vi "SampleSubVI.vi"(0 "task out":refnum<k21> caption="任务输出", 1 "Courter 1":refnum<k21> caption="任务/通道输入1", 3 "Courter 4":refnum<k21> caption="任务/通道输入4", 4 "Courter 2":refnum<k21> caption="任务/通道输入2", 6 "数组":sgl[](array[numeric]), 10 "Courter 3":refnum<k21> caption="任务/通道输入3", 11 "Courter 7":refnum<k21> caption="任务/通道输入7", 15 "Courter 5":refnum<k21> caption="任务/通道输入5", 19 "Courter 8":refnum<k21> caption="任务/通道输入8", 23 "Courter 6":refnum<k21> caption="任务/通道输入6") -> (5 "加速度信号2":dbl[](array[numeric]), 7 "压力信号":dbl[](array[numeric]), 8 "轴向位移":dbl[](array[numeric]), 9 "轴向力":dbl[](array[numeric]), 12 "vmic反馈数据":sgl[](array[numeric]), 13 "力臂":dbl[](array[numeric]), 14 "AngleSample":dbl[](array[numeric]), 16 "加速度信号":dbl[](array[numeric]), 17 "同步信号":dbl[](array[numeric]), 18 "AngleSample 2":dbl[](array[numeric]), 20 "ForceSampledata":dbl[](array[numeric]), 21 "F_outrange":bool[](array[boolean]), 24 "error out":errorcluster, 25 "PositionSampleData":dbl[](array[numeric]), 27 "TorqueSample":dbl[](array[numeric]))   [LabVIEW 2014]
uses:
  <vilib>/DAQmx/read.llb/DAQmx Read (Analog 1D DBL NChan 1Samp).vi
  <vilib>/DAQmx/read.llb/DAQmx Read (Counter DBL 1Chan 1Samp).vi
panel:
  out "ACC1 4":dbl
  out "ACC1 3":dbl
  out "ACC1 2":dbl
  out "ACC1":dbl
  out "data":dbl[](array[numeric]) caption="数据" format="%0.2f"
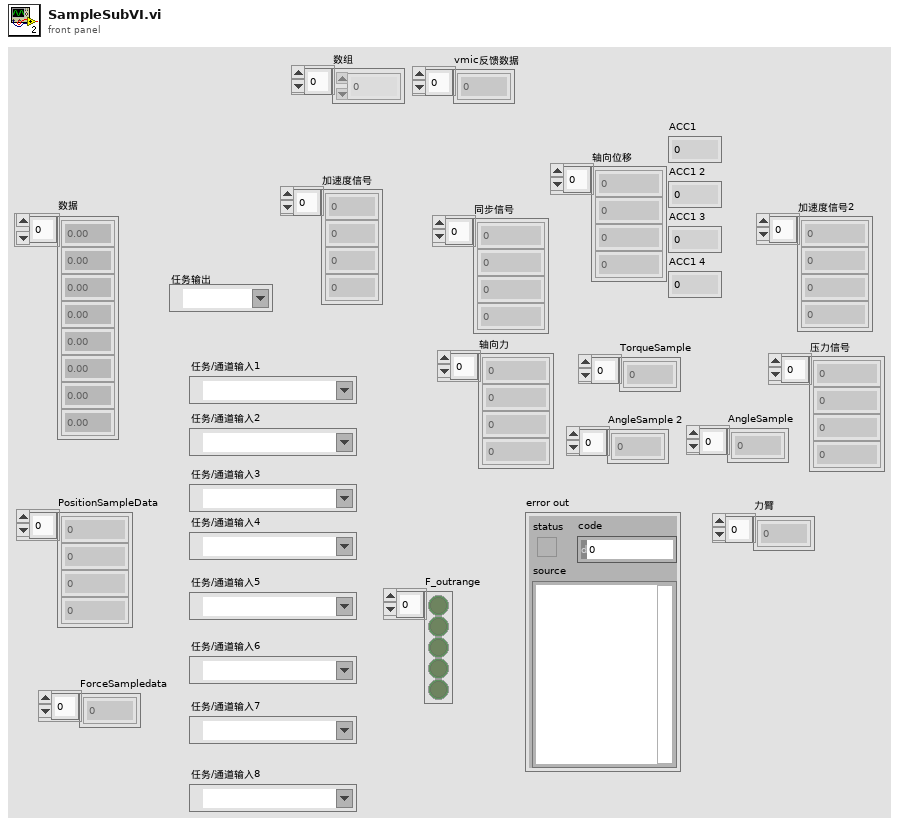
[diagram p1: front panel]
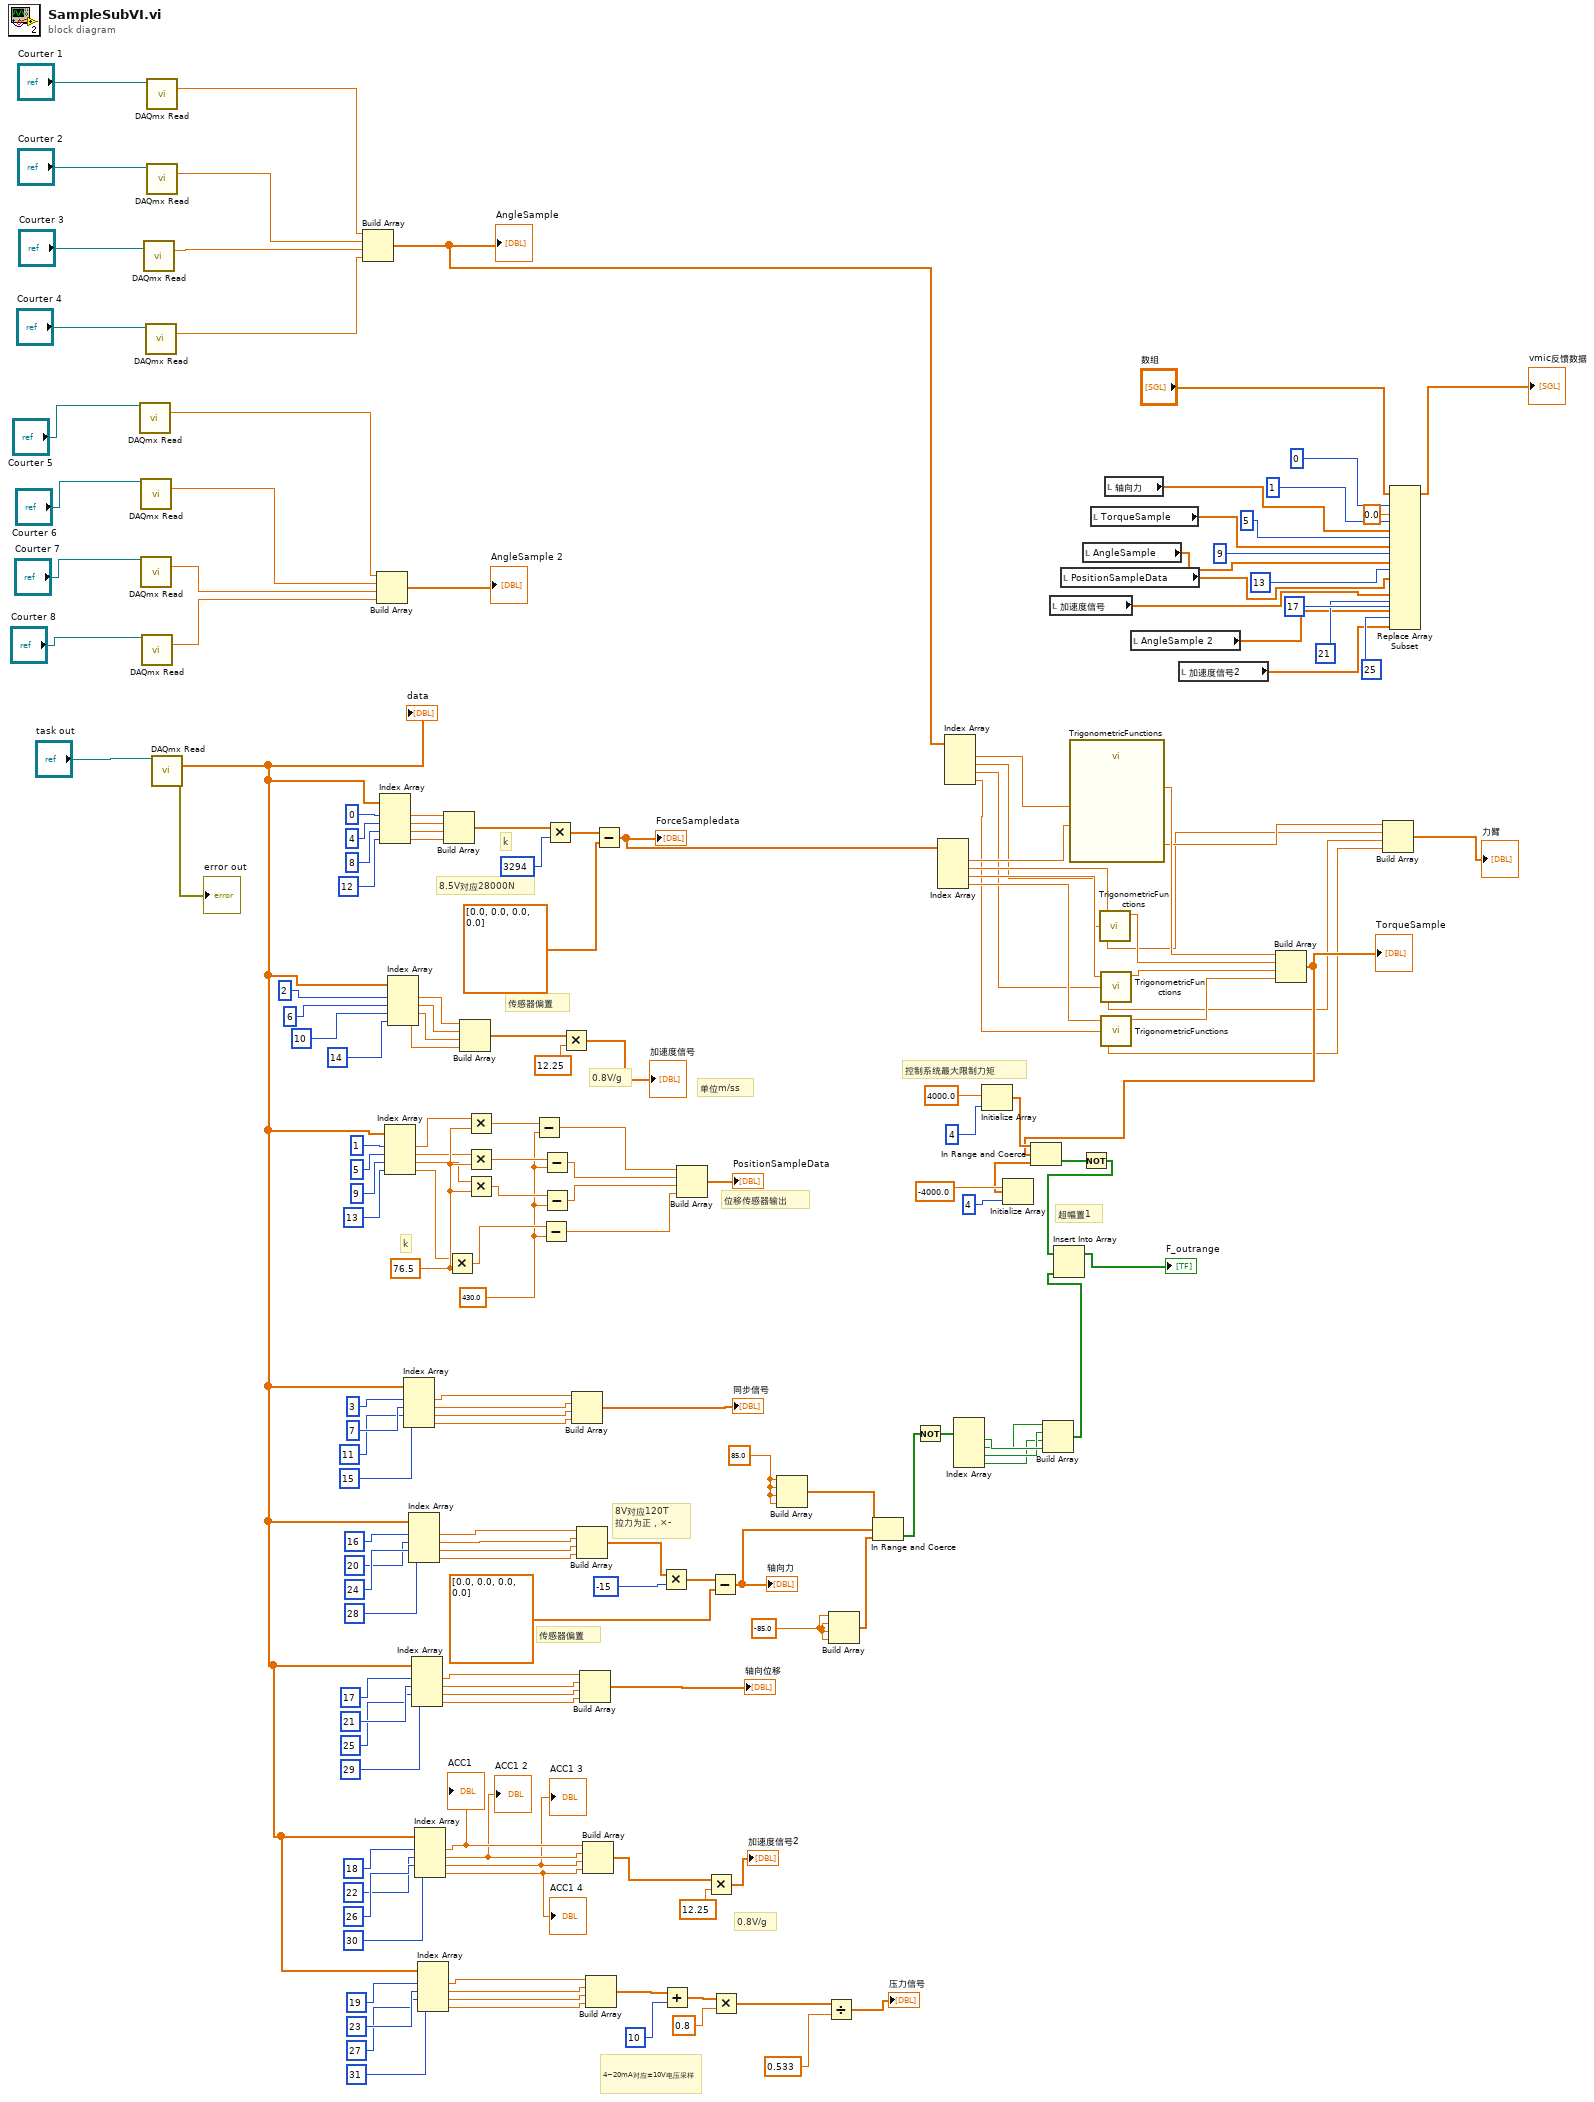
[diagram p0: block diagram]
diagram:
  w68 = -85.0
  w70 = 85.0
  w153 = 430.0 ("y")
  w167 = 76.5 ("y")
  # "0.8V/g"
  # "4~20mA对应±10V电压采样"
  # "单位m/ss"
  # "8V对应120T\n拉力为正，×-"
  # "传感器偏置"
  # "0.8V/g"
  # "位移传感器输出"
  # "超幅置1"
  # "8.5V对应28000N"
  # "k"
  # "k"
  # "控制系统最大限制力矩"
  # "传感器偏置"
  n1 = call-poly <vilib>:"DAQmx Read.vi"("task/channels in"="Courter 5") -> ("data"=w27:dbl)  [unwired: 12 in, 2 out]
  n2 = call-poly <vilib>:"DAQmx Read.vi"("task/channels in"="Courter 6") -> ("data"=w26:dbl)  [unwired: 12 in, 2 out]
  n3 = call-poly <vilib>:"DAQmx Read.vi"("task/channels in"="Courter 7") -> ("data"=w25:dbl)  [unwired: 12 in, 2 out]
  n4 = call-poly <vilib>:"DAQmx Read.vi"("task/channels in"="Courter 8") -> ("data"=w24:dbl)  [unwired: 12 in, 2 out]
  n5 = call-poly <vilib>:"DAQmx Read.vi"("task/channels in"="Courter 3") -> ("data"=w19:dbl)  [unwired: 12 in, 2 out]
  n6 = call-poly <vilib>:"DAQmx Read.vi"("task/channels in"="Courter 4") -> ("data"=w48:dbl)  [unwired: 12 in, 2 out]
  n7 = call-poly <vilib>:"DAQmx Read.vi"("task/channels in"="Courter 1") -> ("data"=w50:dbl)  [unwired: 12 in, 2 out]
  n8 = call-poly <vilib>:"DAQmx Read.vi"("task/channels in"="Courter 2") -> ("data"=w49:dbl)  [unwired: 12 in, 2 out]
  n9 = call-poly <vilib>:"DAQmx Read.vi"("task/channels in"="task out") -> ("data"=w97:dbl[], "error out"=→"error out":errorcluster)  [unwired: 12 in, 1 out]
  "data" <- w97
  n10 = Build Array(w50, w49, w19, w48) -> (w47:dbl[])
  "AngleSample" <- w47
  n11 = Build Array(w27, w26, w25, w24) -> (→"AngleSample 2":dbl[])
  n12 = Index Array(array=w97, index #1=0 ("索引"), index #2=4 ("索引"), index #3=8 ("索引"), index #4=12 ("索引")) -> (element #1=w88:dbl, element #2=w86:dbl, element #3=w158:dbl, element #4=w171:dbl)
  n13 = Index Array(array=w97, index #1=1 ("索引"), index #2=5 ("索引"), index #3=9 ("索引"), index #4=13 ("索引")) -> (element #1=w162:dbl, element #2=w161:dbl, element #3=w160:dbl, element #4=w159:dbl)
  n14 = Index Array(array=w97, index #1=2 ("索引"), index #2=6 ("索引"), index #3=10 ("索引"), index #4=14 ("索引")) -> (element #1=w146:dbl, element #2=w145:dbl, element #3=w144:dbl, element #4=w143:dbl)
  n15 = Index Array(array=w97, index #1=3 ("索引"), index #2=7 ("索引"), index #3=11 ("索引"), index #4=15 ("索引")) -> (element #1=w136:dbl, element #2=w135:dbl, element #3=w134:dbl, element #4=w133:dbl)
  n16 = Index Array(array=w97, index #1=16 ("索引"), index #2=20 ("索引"), index #3=24 ("索引"), index #4=28 ("索引")) -> (element #1=w41:dbl, element #2=w42:dbl, element #3=w130:dbl, element #4=w131:dbl)
  n17 = Index Array(array=w97, index #1=17 ("索引"), index #2=21 ("索引"), index #3=25 ("索引"), index #4=29 ("索引")) -> (element #1=w125:dbl, element #2=w124:dbl, element #3=w123:dbl, element #4=w122:dbl)
  n18 = Index Array(array=w97, index #1=18 ("索引"), index #2=22 ("索引"), index #3=26 ("索引"), index #4=30 ("索引")) -> (element #1=w106:dbl, element #2=w92:dbl, element #3=w91:dbl, element #4=w90:dbl)
  "ACC1" <- w106
  "ACC1 2" <- w92
  "ACC1 3" <- w91
  "ACC1 4" <- w90
  n19 = Index Array(array=w97, index #1=19 ("索引"), index #2=23 ("索引"), index #3=27 ("索引"), index #4=31 ("索引")) -> (element #1=w105:dbl, element #2=w104:dbl, element #3=w103:dbl, element #4=w102:dbl)
  n20 = Build Array(w88, w86, w158, w171) -> (w170:dbl[])
  n21 = Multiply(x=w159, y=w167) -> (x*y=w154:dbl)
  n22 = Build Array(w146, w145, w144, w143) -> (w147:dbl[])
  n23 = Multiply(x=w162, y=w167) -> (x*y=w157:dbl)
  n24 = Multiply(x=w161, y=w167) -> (x*y=w156:dbl)
  n25 = Multiply(x=w160, y=w167) -> (x*y=w155:dbl)
  n26 = Subtract(x=w157, y=w153) -> (x-y=w87:dbl)
  n27 = Subtract(x=w154, y=w153) -> (x-y=w89:dbl)
  n28 = Subtract(x=w156, y=w153) -> (x-y=w85:dbl)
  n29 = Subtract(x=w155, y=w153) -> (x-y=w152:dbl)
  n30 = Multiply(x=w170, y=3294) -> (x*y=w177:dbl[])
  n31 = Multiply(x=w147, y=12.25) -> (x*y=→"加速度信号":dbl[])
  n32 = Build Array(w136, w135, w134, w133) -> (→"同步信号":dbl[])
  n33 = Build Array(w41, w42, w130, w131) -> (w112:dbl[])
  n34 = Build Array(w125, w124, w123, w122) -> (→"轴向位移":dbl[])
  n35 = Build Array(w106, w92, w91, w90) -> (w21:dbl[])
  n36 = Build Array(w105, w104, w103, w102) -> (w45:dbl[])
  n37 = Subtract(x=w177, y=dbl[] [0.0, 0.0, 0.0, 0.0]) -> (x-y=w84:dbl[])
  "ForceSampledata" <- w84
  n38 = Multiply(x=w112, y=-15) -> (x*y=w114:dbl[])
  n39 = Add(x=w45, y=10) -> (x+y=w39:dbl[])
  n40 = Build Array(w87, w85, w152, w89) -> (→"PositionSampleData":dbl[])
  n41 = Multiply(x=w21, y=12.25) -> (x*y=→"加速度信号2":dbl[])
  n42 = Subtract(x=w114, y=dbl[] [0.0, 0.0, 0.0, 0.0]) -> (x-y=w96:dbl[])
  "轴向力" <- w96
  n43 = Multiply(x=w39, y=0.8) -> (x*y=w38:dbl[])
  n44 = Build Array(w70, w70, w70, w70) -> (w69:dbl[])
  n45 = Divide(x=w38, y=0.533) -> (x/y=→"压力信号":dbl[])
  n46 = Build Array(w68, w68, w68, w68) -> (w67:dbl[])
  n47 = In Range and Coerce(upper limit=w69, x=w96, lower limit=w67) -> (In Range?=w95:bool[])  [unwired: 1 out]
  n48 = Not(x=w95) -> (.not. x?=w66:bool[])
  n49 = Index Array(array=w84) -> (element #1=w83:dbl, element #2=w82:dbl, element #3=w81:dbl, element #4=w80:dbl)  [unwired: 4 in]
  n50 = Index Array(array=w47) -> (element #1=w78:dbl, element #2=w77:dbl, element #3=w76:dbl, element #4=w75:dbl)  [unwired: 4 in]
  n51 = Index Array(array=w66) -> (element #1=w65:bool, element #2=w64:bool, element #3=w63:bool, element #4=w62:bool)  [unwired: 4 in]
  n52 = Initialize Array(4000.0, 4) -> (w59:dbl[])
  n53 = Initialize Array(-4000.0, 4) -> (w55:dbl[])
  n54 = Build Array(w64, w63, w62, w65) -> (w61:bool[])
  n55 = local read "加速度信号"() -> (w6:dbl[])
  n56 = local read "PositionSampleData"() -> (w7:dbl[])
  n57 = call "TrigonometricFunctions.vi"("摆角采样"=w78, "力采样N"=w83) -> ("力矩采样Nm"=w74:dbl, "力臂"=w36:dbl)  [unwired: 5 in]
  n58 = local read "AngleSample"() -> (w8:dbl[])
  n59 = local read "TorqueSample"() -> (w9:dbl[])
  n60 = call "TrigonometricFunctions.vi"("摆角采样"=w77, "力采样N"=w82) -> ("力矩采样Nm"=w73:dbl, "力臂"=w35:dbl)  [unwired: 5 in]
  n61 = call "TrigonometricFunctions.vi"("摆角采样"=w76, "力采样N"=w81) -> ("力矩采样Nm"=w72:dbl, "力臂"=w34:dbl)  [unwired: 5 in]
  n62 = call "TrigonometricFunctions.vi"("摆角采样"=w75, "力采样N"=w80) -> ("力矩采样Nm"=w71:dbl, "力臂"=w33:dbl)  [unwired: 5 in]
  n63 = local read "轴向力"() -> (w10:dbl[])
  n64 = local read "AngleSample 2"() -> (w5:dbl[])
  n65 = local read "加速度信号2"() -> (w4:dbl[])
  n66 = Build Array(w74, w73, w72, w71) -> (w37:dbl[])
  "TorqueSample" <- w37
  n67 = In Range and Coerce(upper limit=w59, x=w37, lower limit=w55) -> (In Range?=w169:bool[])  [unwired: 1 out]
  n68 = Not(x=w169) -> (.not. x?=w94:bool[])
  n69 = Insert Into Array(array=w94, new element=w61) -> (→"F_outrange":bool[])  [unwired: 1 in]
  n70 = Build Array(w36, w35, w34, w33) -> (→"力臂":dbl[])
  n71 = Replace Array Subset(array="数组", new element #1=sgl 0.0 ("新元素/子数组"), index #1=0 ("索引"), new element #2=w10, index #2=1 ("索引"), new element #3=w9, index #3=5 ("索引"), new element #4=w8, index #4=9 ("索引"), new element #5=w7, index #5=13 ("索引"), new element #6=w6, index #6=17 ("索引"), new element #7=w5, index #7=21 ("索引"), new element #8=w4, index #8=25 ("索引")) -> (→"vmic反馈数据":sgl[])
